vi "Plus Minus Correction.vi"(0 "string":string) -> (1 "plusminus":bool, 2 "new string":string)   [LabVIEW 2017, in "NI_Gmath.lvlib"]
uses:
  NI_Gmath.lvlib
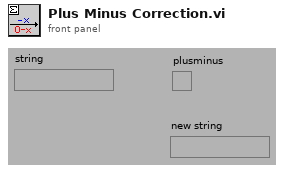
[diagram p1: front panel]
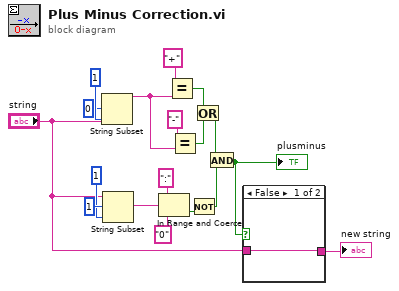
[diagram p0: block diagram]
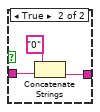
[diagram p2: hidden frame]
diagram:
  n1 = String Subset(string="string", offset (0)=0, length (rest)=1) -> (substring=w12:string)
  n2 = String Subset(string="string", offset (0)=1, length (rest)=1) -> (substring=w8:string)
  n3 = In Range and Coerce(upper limit=":", x=w8, lower limit="0") -> (In Range?=w4:bool)  [unwired: 1 out]
  n4 = Equal?(x="+", y=w12) -> (x = y?=w11:bool)
  n5 = Equal?(x="-", y=w12) -> (x = y?=w10:bool)
  n6 = Not(x=w4) -> (.not. x?=w5:bool)
  n7 = Or(x=w11, y=w10) -> (x .or. y?=w6:bool)
  n8 = And(x=w6, y=w5) -> (x .and. y?=w1:bool)
  "plusminus" <- w1
  n9 = case shown="False" w1 {
    tunnel: [w19 w22] -> w2
    tunnel: "string" -> [w19 w21]
    frame False {
    }
    frame True {
      n10 = Concatenate Strings("0", w21) -> (w22:string)
    }
  }
  "new string" <- w2
